vi "Build.Auto Build Manager.vi"(11 "App Build Spec":u16(ring) items=["Circle Test App", "Circle Test App Installer"]) -> (0 "Error":errorcluster, 3 "Build Ver":string)   [LabVIEW 2018]
uses:
  <vilib>/AppBuilder/AB_API_Simple/Get Build Specification Version (project reference).vi
  <vilib>/AppBuilder/AB_API_Simple/Build (project reference).vi
  <vilib>/Utility/config.llb/Write Key (Boolean).vi
  <vilib>/AppBuilder/AB_API_Simple/NI_App_Builder_API.lvlib
  <vilib>/KATE/Files/File Utils.lvlib
  <vilib>/Utility/config.llb/NI_LVConfig.lvlib
panel:
  in  "Proj List refresh":bool
  in  "Project":i32(ring) items=["Circle Test.lvproj"]
  out "MultInst":string
  in  "MultExe":bool caption="Allow Multiple Exe Instances"
  in  "Open Installer Folder":bool
  out "Found Installer":bool
  out "Status":string
  in  "Clear Error":bool
  in  "Exit":bool
  in  "Build":bool
  in  "Build Installer":bool=TRUE
  in  "Build App":bool=TRUE
  out "Building Installer":bool
  out "Building App":bool
  in  "Data Tab":T1(tab)
  out "App files":path[](array[path])
  out "Installer files":path[](array[path])
  out "New Path":path
  out "Orig Path":path
  out "BuildSpecs":string[](array[string])
  out "BuildDir":path
  out "BuildINI":path
  in  "Installer Build Spec":string
  # "App Builder"
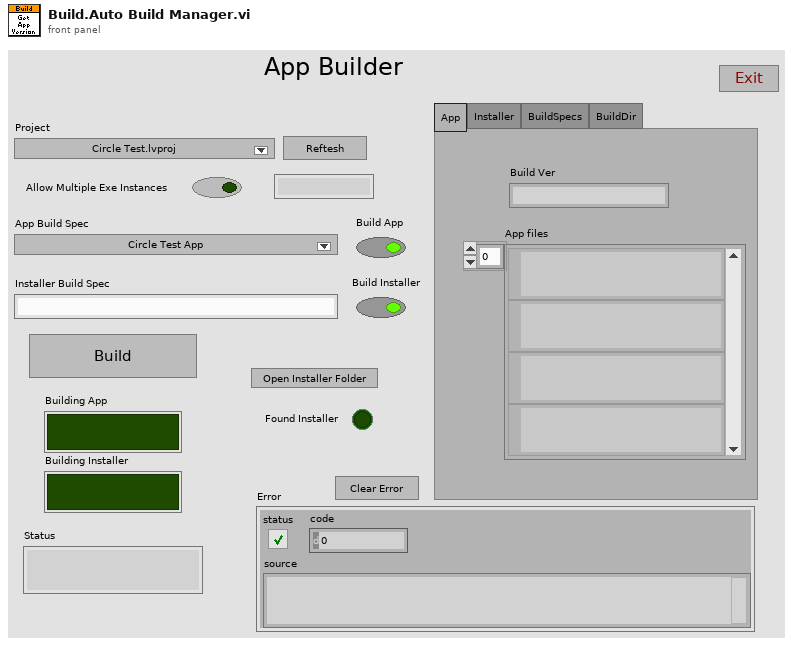
[diagram p1: front panel]
types:
  T1 = enum32{"App", "Installer", "BuildSpecs", "BuildDir"}
  T2 = cluster{"Proj":refnum<vi>, "Proj Name":string, "App Ver":string, "Installer":refnum<vi>, "Installer Name":string, "BuildSpec":refnum<vi>}
  T3 = typedef "NI_App_Builder_API.lvlib/Build Specification Version.ctl" = cluster{"Major":u16, "Minor":u16, "Fix":u16, "Build":u16}
  T4 = typedef "NI_LVConfig.lvlib/Config Data RefNum.ctl" = refnum<k1>
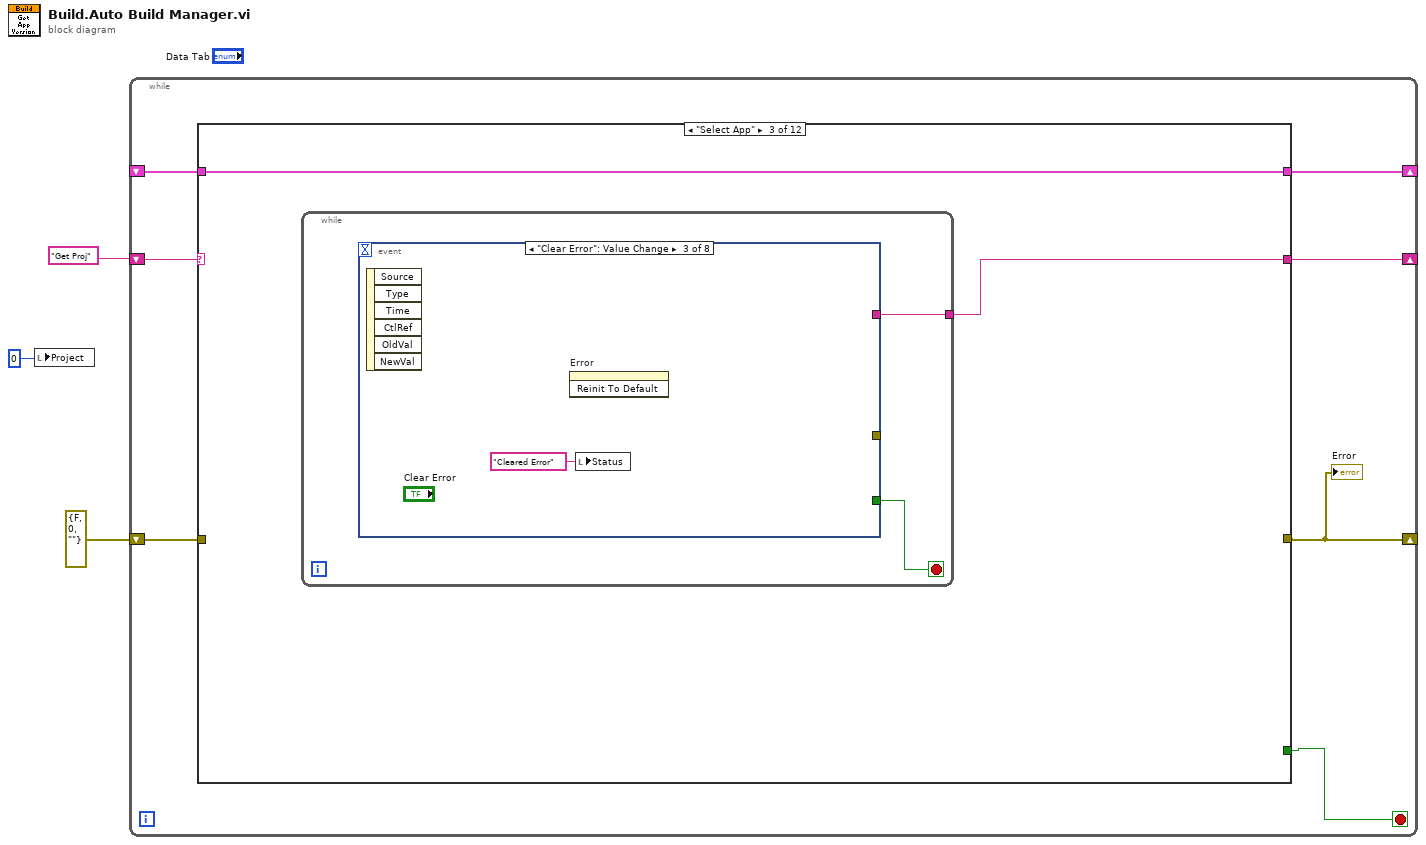
[diagram p0: block diagram]
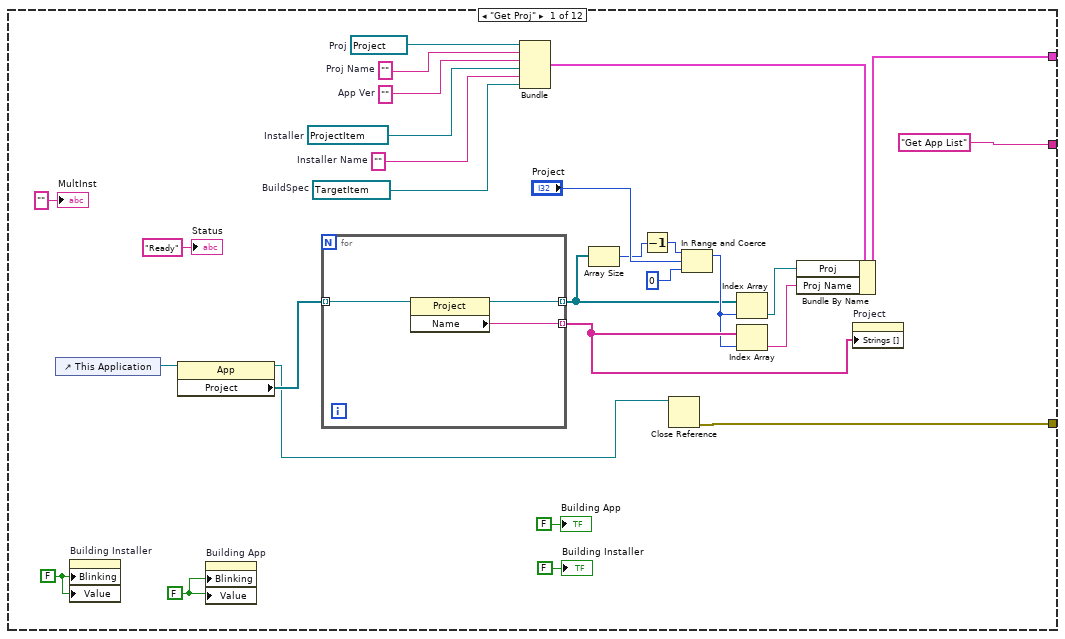
[diagram p2: hidden frame]
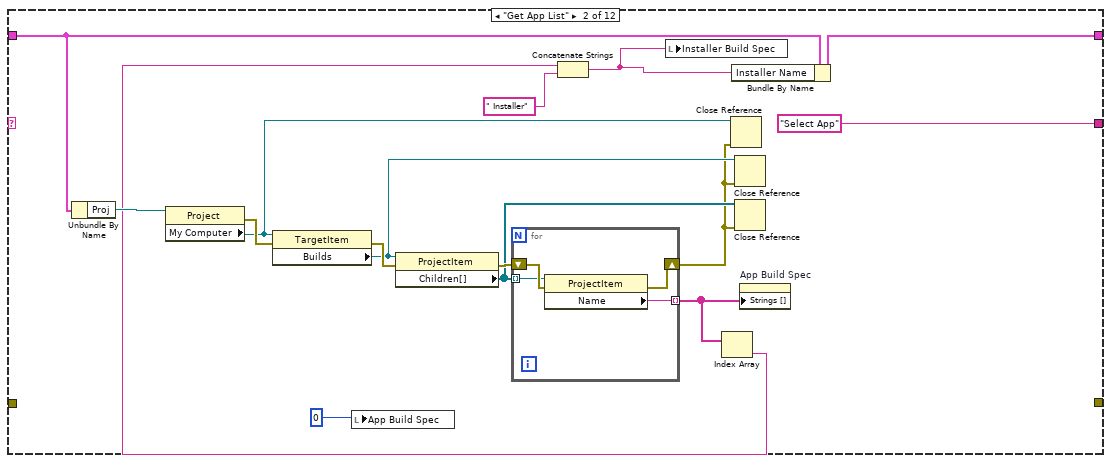
[diagram p3: hidden frame]
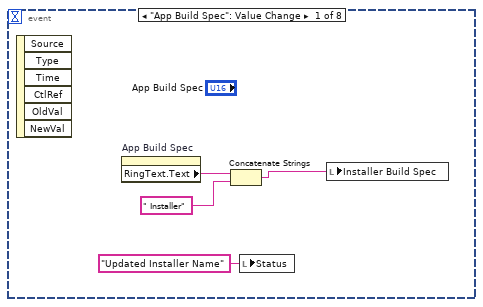
[diagram p4: hidden frame]
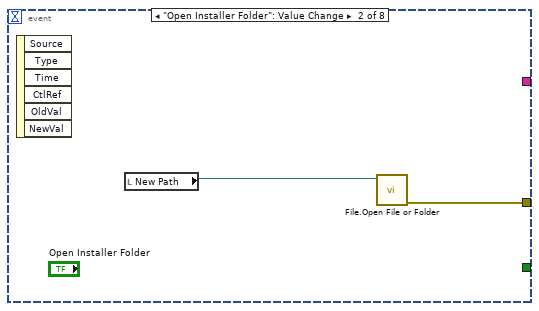
[diagram p5: hidden frame]
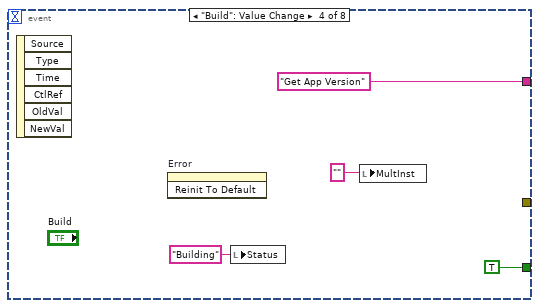
[diagram p6: hidden frame]
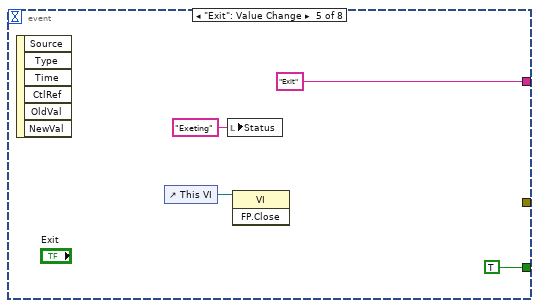
[diagram p7: hidden frame]
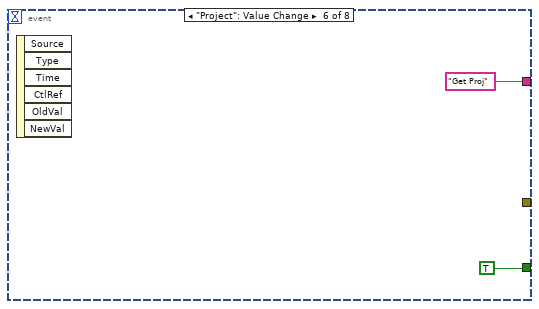
[diagram p8: hidden frame]
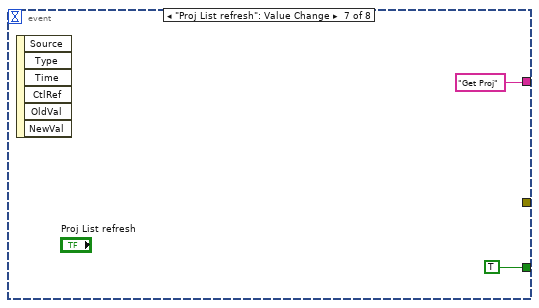
[diagram p9: hidden frame]
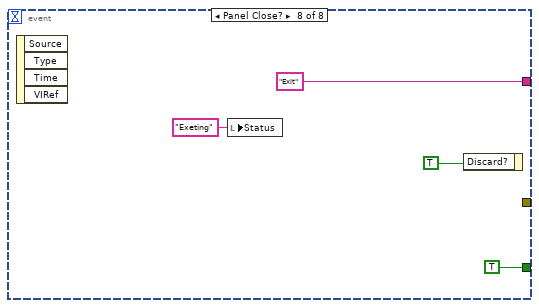
[diagram p10: hidden frame]
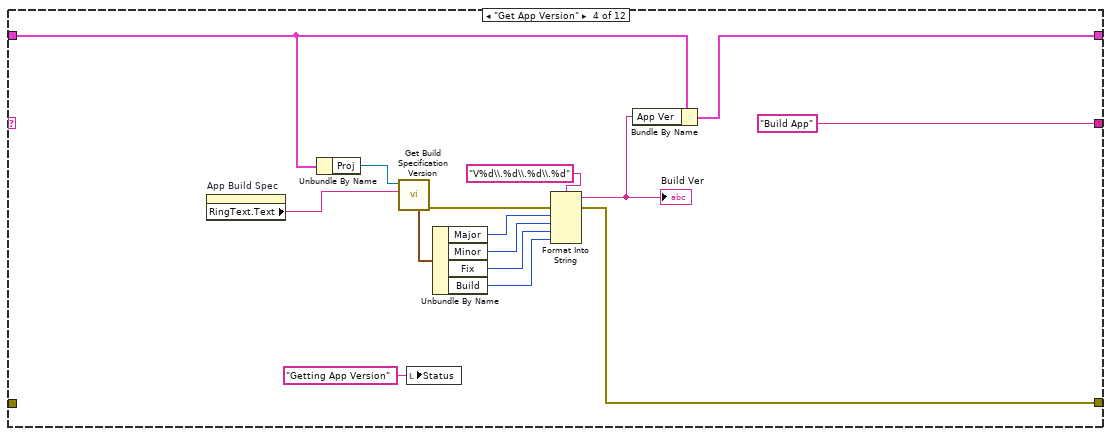
[diagram p11: hidden frame]
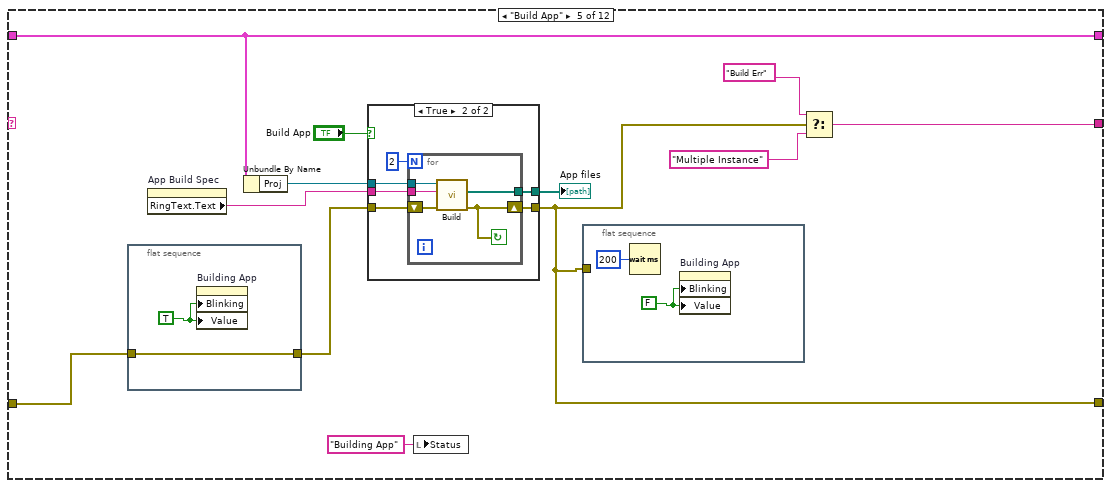
[diagram p12: hidden frame]
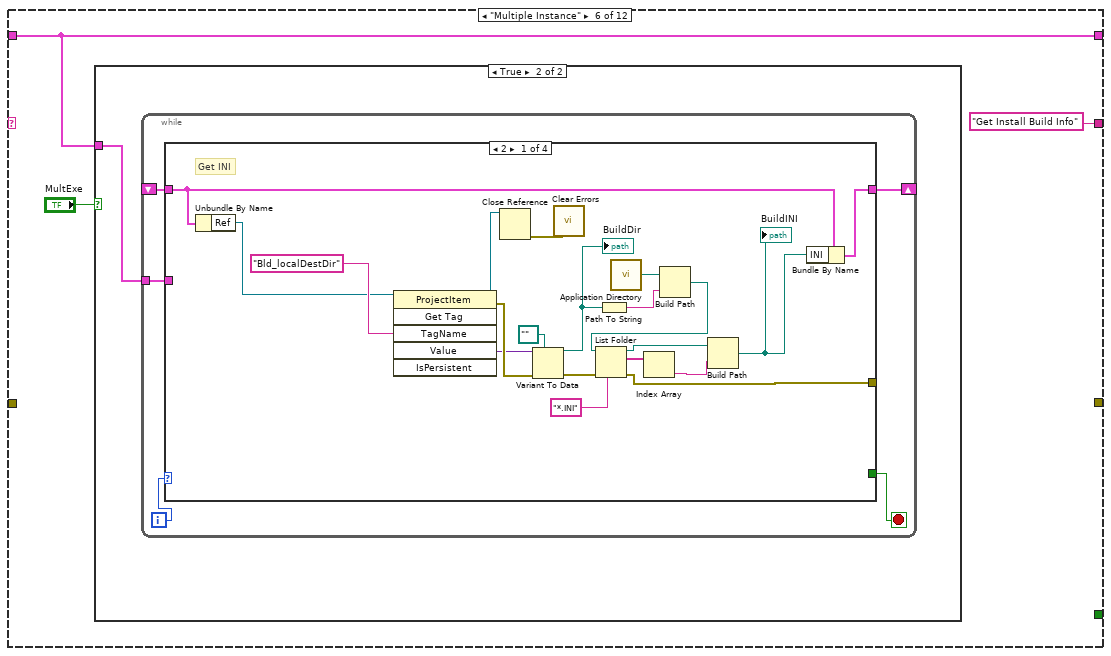
[diagram p14: hidden frame]
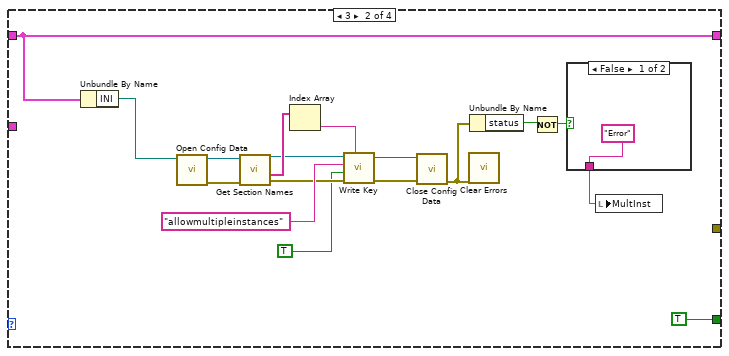
[diagram p16: hidden frame]
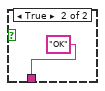
[diagram p17: hidden frame]
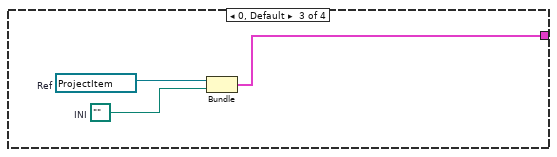
[diagram p18: hidden frame]
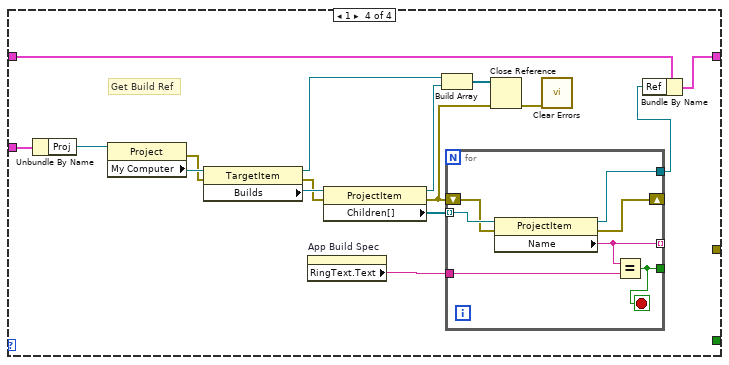
[diagram p19: hidden frame]
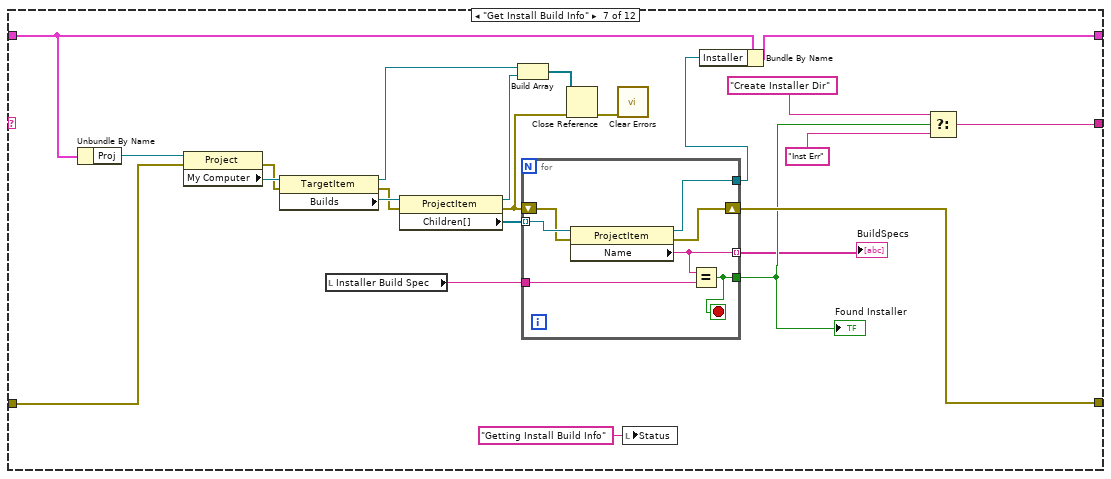
[diagram p20: hidden frame]
diagram:
  n1 = local write "Project"(0) -> ()
  n2 = while {
    shift-right: [w8] -> _
    shift-left: _ -> [w9]
    shift-right: [w7] -> _
    shift-left: "Get Proj" -> [w10]
    shift-right: [w5] -> _
    shift-left: errorcluster {"status"=FALSE, "code"=0, "source"=""} ("error constant") -> [w6]
    stop <- w4 stop-if-true
    n3 = case shown="\"Select App\"" w10 {
      tunnel: w9 -> [_ w44 w63 w95 w114 w132 w215 w238 w241 w256 w263 w284]
      tunnel: [w33 w43 w63 w93 w114 w132 w214 w238 w241 w256 w263 _] -> w8
      tunnel: ["Get App List" "Select App" w62 "Build App" w107 "Get Install Build Info" w210 "Select App" "Select App" "Build Installer" "Select App" _] -> w7
      tunnel: [w31 _ _ w89 w105 _ w221 errorcluster {"status"=TRUE, "code"=1, "source"="Installer not found.  Check Name."} ("error constant") errorcluster {"status"=TRUE, "code"=1, "source"="Build Error."} ("error constant") w242 w262 _] -> w5
      tunnel: w6 -> [_ _ _ _ w112 _ w224 _ _ _ _ _]
      tunnel: [_ _ _ _ _ _ _ _ _ _ _ TRUE] -> w4
      frame "Get Proj" {
        w22 = FALSE ("Building App")
        w23 = FALSE ("Blinking")
        w25 = refnum<vi> refnum  # BuildSpec
        w27 = refnum<vi> refnum  # Installer
        w28 = ""  # Installer Name
        w32 = ""  # App Ver
        w36 = refnum<vi> refnum  # Proj
        w37 = ""  # Proj Name
        n4 = control-ref of="This Application"() -> (w38:refnum<vi>)
        n5 = property on="Building Installer" class="Bool (strict)"("Blinking"=w23, "Value"=w23) -> ()  [unwired: 2 in, 2 out]
        n6 = property class="App"(reference=w38) -> (reference out=w20:refnum<vi>, "Project"=w21:refnum<vi>[])  [unwired: 1 in, 1 out]
        n7 = property on="Building App" class="Bool (strict)"("Blinking"=w22, "Value"=w22) -> ()  [unwired: 2 in, 2 out]
        n8 = for {
          tunnel: w21 -> [w41] mode=indexing
          tunnel: [w40] -> w17 mode=indexing
          tunnel: [w39] -> w14 mode=indexing
          n9 = property class="Project"(reference=w41) -> (reference out=w39:refnum<vi>, "Name"=w40:string)  [unwired: 1 in, 1 out]
        }
        n10 = Bundle("Proj"=w36, "Proj Name"=w37, "App Ver"=w32, "Installer"=w27, "Installer Name"=w28, "BuildSpec"=w25) -> (w34:T2)  [unwired: 1 in]
        n11 = Array Size(array=w14) -> (size(s)=w12:i32)
        n12 = Decrement(x=w12) -> (x-1=w11:i32)
        n13 = Close Reference(reference=w20) -> (error out=w31:errorcluster)  [unwired: 1 in]
        n14 = In Range and Coerce(upper limit=w11, x="Project", lower limit=0) -> (coerced(x)=w15:i32)  [unwired: 1 out]
        n15 = Index Array(array=w14, index=w15) -> (element=w19:refnum<vi>)
        n16 = Index Array(array=w17, index=w15) -> (element=w18:string)
        n17 = Bundle By Name(cluster=w34, "Proj"=w19, "Proj Name"=w18) -> (w33:T2)
        n18 = property on="Project" class="Ring (strict)"("Strings []"=w17) -> ()  [unwired: 2 in, 2 out]
        "Building App" <- FALSE ("Building App")
        "Building Installer" <- FALSE ("Building Installer")
        "Status" <- "Ready" ("Status")
        "MultInst" <- "" ("MultInst")
      }
      frame "Get App List" {
        n19 = Unbundle By Name(w44) -> ("Proj"=w57:refnum<vi>)
        n20 = property class="Project"(reference=w57) -> (error out=w56:errorcluster, "My Computer"=w51:refnum<vi>)  [unwired: 1 in, 1 out]
        n21 = property class="TargetItem"(reference=w51, error in=w56) -> (error out=w55:errorcluster, "Builds"=w52:refnum<vi>)  [unwired: 1 out]
        n22 = local write "App Build Spec"(u16 0) -> ()
        n23 = property class="ProjectItem"(reference=w52, error in=w55) -> (error out=w54:errorcluster, "Children[]"=w53:refnum<vi>[])  [unwired: 1 out]
        n24 = for {
          shift-right: [w59] -> w50
          shift-left: w54 -> [w61]
          tunnel: w53 -> [w60] mode=indexing
          tunnel: [w58] -> w48 mode=indexing
          n25 = property class="ProjectItem"(reference=w60, error in=w61) -> (error out=w59:errorcluster, "Name"=w58:string)  [unwired: 1 out]
        }
        n26 = Index Array(array=w48) -> (element=w46:string)  [unwired: 1 in]
        n27 = Concatenate Strings(w46, " Installer") -> (w42:string)
        n28 = local write "Installer Build Spec"(w42) -> ()
        n29 = Close Reference(reference=w51, error in (no error)=w50) -> ()  [unwired: 1 out]
        n30 = Bundle By Name(cluster=w44, "Installer Name"=w42) -> (w43:T2)
        n31 = Close Reference(reference=w52, error in (no error)=w50) -> ()  [unwired: 1 out]
        n32 = Close Reference(reference=w53, error in (no error)=w50) -> ()  [unwired: 1 out]
        n33 = property on="App Build Spec" class="Ring (strict)"("Strings []"=w48) -> ()  [unwired: 2 in, 2 out]
      }
      frame "Select App" {
        n34 = while {
          tunnel: [w65] -> w62
          stop <- w64 stop-if-true
          n35 = event shown="[2] \"Clear Error\": Value Change" {
            selector: _ -> [_ _ _ _ _ _ _ _]
            dyn-events: _ -> [_ _ _ _ _ _ _ _]
            timeout: _ -> [_ _ _ _ _ _ _ _]
            tunnel: [_ _ _ "Get App Version" "Exit" "Get Proj" "Get Proj" "Exit"] -> w65
            tunnel: [_ _ _ TRUE TRUE TRUE TRUE TRUE] -> w64
            tunnel: [_ w71 _ _ _ _ _ _] -> _
            event "App Build Spec": Value Change {
              n36 = event-data() -> ()  [unwired: 1 in, 6 out]
              n37 = property on="App Build Spec" class="Ring (strict)"() -> ("RingText.Text"=w69:string)  [unwired: 2 in, 2 out]
              n38 = Concatenate Strings(w69, " Installer") -> (w68:string)
              n39 = local write "Status"("Updated Installer Name" ("Status")) -> ()
              n40 = local write "Installer Build Spec"(w68) -> ()
            }
            event "Open Installer Folder": Value Change {
              n41 = event-data() -> ()  [unwired: 1 in, 6 out]
              n42 = local read "New Path"() -> (w70:path)
              n43 = call <vilib>:"File.Open File or Folder.vi"("Path"=w70) -> ("Error Out"=w71:errorcluster)  [unwired: 10 in]
            }
            event "Clear Error": Value Change {
              n44 = event-data() -> ()  [unwired: 1 in, 6 out]
              n45 = invoke on="Error" class="Clust (strict)" method="Reinit To Default"() -> ()  [unwired: 3 in, 3 out]
              n46 = local write "Status"("Cleared Error" ("Status")) -> ()
            }
            event "Build": Value Change {
              n47 = event-data() -> ()  [unwired: 1 in, 6 out]
              n48 = invoke on="Error" class="Clust (strict)" method="Reinit To Default"() -> ()  [unwired: 3 in, 3 out]
              n49 = local write "Status"("Building" ("Status")) -> ()
              n50 = local write "MultInst"("" ("MultInst")) -> ()
            }
            event "Exit": Value Change {
              n51 = event-data() -> ()  [unwired: 1 in, 6 out]
              n52 = control-ref of="This VI"() -> (w77:refnum<vi>)
              n53 = local write "Status"("Exeting" ("Status")) -> ()
              n54 = invoke class="VI" method="FP.Close"(reference=w77) -> ()  [unwired: 2 in, 3 out]
            }
            event "Project": Value Change {
              n55 = event-data() -> ()  [unwired: 1 in, 6 out]
            }
            event "Proj List refresh": Value Change {
              n56 = event-data() -> ()  [unwired: 1 in, 6 out]
            }
            event Panel Close? {
              n57 = event-data() -> ()  [unwired: 1 in, 4 out]
              n58 = local write "Status"("Exeting" ("Status")) -> ()
              n59 = event-data("Discard?"=TRUE) -> ()  [unwired: 1 in, 1 out]
            }
          }
        }
      }
      frame "Get App Version" {
        n60 = property on="App Build Spec" class="Ring (strict)"() -> ("RingText.Text"=w91:string)  [unwired: 2 in, 2 out]
        n61 = Unbundle By Name(w95) -> ("Proj"=w96:refnum<vi>)
        n62 = call-poly <vilib>:"Get Build Specification Version.vi"("Name of build specification"=w91, "Project reference"=w96) -> ("error out"=w103:errorcluster, "Build Specification Version"=w99:T3)  [unwired: 7 in, 1 out]
        n63 = local write "Status"("Getting App Version" ("Status")) -> ()
        n64 = Unbundle By Name(w99) -> ("Major"=w100:u16, "Minor"=w101:u16, "Fix"=w102:u16, "Build"=w97:u16)
        n65 = Format Into String(format string="V%d\\.%d\\.%d\\.%d", error in=w103, w100, w101, w102, w97) -> (resulting string=w94:string, error out=w89:errorcluster)  [unwired: 1 in]
        "Build Ver" <- w94
        n66 = Bundle By Name(cluster=w95, "App Ver"=w94) -> (w93:T2)
      }
      frame "Build App" {
        n67 = flat-sequence {
          tunnel: w112 -> [w130]
          tunnel: [w130] -> w111
          frame #0 {
            w131 = TRUE ("Building App")
            n68 = property on="Building App" class="Bool (strict)"("Blinking"=w131, "Value"=w131) -> ()  [unwired: 2 in, 2 out]
          }
        }
        n69 = property on="App Build Spec" class="Ring (strict)"() -> ("RingText.Text"=w109:string)  [unwired: 2 in, 2 out]
        n70 = Unbundle By Name(w114) -> ("Proj"=w115:refnum<vi>)
        n71 = case shown="True" "Build App" {
          tunnel: w115 -> [_ w122]
          tunnel: w109 -> [_ w121]
          tunnel: [_ w120] -> w113
          tunnel: [w116 w119] -> w105
          tunnel: w111 -> [w116 w118]
          frame False {
          }
          frame True {
            n72 = for {
              N: 2 -> [_]
              tunnel: w122 -> [w127]
              tunnel: w121 -> [w126]
              tunnel: [w125] -> w120
              shift-right: [w123] -> w119
              shift-left: w118 -> [w124]
              stop <- w123 continue-if-true
              n73 = call-poly <vilib>:"Build.vi"("error in (no error)"=w124, "Name of build specification (if empty: build all)"=w126, "Project reference"=w127) -> ("error out"=w123:errorcluster, "Generated files"=w125:path[])  [unwired: 6 in, 1 out]
            }
          }
        }
        "App files" <- w113
        n74 = local write "Status"("Building App" ("Status")) -> ()
        n75 = flat-sequence {
          tunnel: w105 -> [_]
          frame #0 {
            w129 = FALSE ("Building App")
            n76 = Wait (ms)(milliseconds to wait=u32 200) -> ()  [unwired: 1 out]
            n77 = property on="Building App" class="Bool (strict)"("Blinking"=w129, "Value"=w129) -> ()  [unwired: 2 in, 2 out]
          }
        }
        n78 = Select(t="Build Err", s=w105, f="Multiple Instance") -> (s? t:f=w107:string)
      }
      frame "Multiple Instance" {
        n79 = case shown="True" "MultExe" {
          tunnel: w132 -> [_ w135]
          frame False {
          }
          frame True {
            n80 = while {
              shift-right: [w140] -> _
              shift-left: _ -> [w138]
              tunnel: w135 -> [w136]
              i -> [w139]
              stop <- w137 stop-if-true
              n81 = case shown="2" w139 {
                tunnel: [w149 w166 w180 w185] -> w140
                tunnel: w138 -> [w150 w166 _ w186]
                tunnel: [_ TRUE _ _] -> w137
                tunnel: w136 -> [_ _ _ w184]
                tunnel: [w147 _ _ _] -> _
                frame 2 {
                  # "Get INI"
                  n82 = Unbundle By Name(w150) -> ("Ref"=w152:refnum<vi>)
                  n83 = invoke class="ProjectItem" method="Get Tag"(reference=w152, "TagName"="Bld_localDestDir") -> (reference out=w145:refnum<vi>, error out=w160:errorcluster, "Value"=w159:variant)  [unwired: 4 in, 3 out]
                  n84 = Close Reference(reference=w145) -> (error out=w151:errorcluster)  [unwired: 1 in]
                  n85 = Variant To Data(error in=w160, type=path "", Variant=w159) -> (data=w143:path, error out=w148:errorcluster)
                  "BuildDir" <- w143
                  n86 = call <vilib>:"Clear Errors.vi"("error in (no error)"=w151) -> ()  [unwired: 5 in, 2 out]
                  n87 = Path To String(path=w143) -> (string=w142:string)
                  n88 = call <vilib>:"Application Directory.vi"() -> ("Application Directory"=w144:path)
                  n89 = Build Path(base path=w144, name or relative path=w142) -> (appended path=w141:path)
                  n90 = List Folder(path=w141, pattern="*.INI", error in=w148) -> (path out=w154:path, filenames=w155:string[], error out=w147:errorcluster)  [unwired: 1 in, 1 out]
                  n91 = Index Array(array=w155) -> (element=w153:string)  [unwired: 1 in]
                  n92 = Build Path(base path=w154, name or relative path=w153) -> (appended path=w146:path)
                  "BuildINI" <- w146
                  n93 = Bundle By Name(cluster=w150, "INI"=w146) -> (w149:cluster{"Ref":refnum<vi>, "INI":path})
                }
                frame 3 {
                  n94 = Unbundle By Name(w166) -> ("INI"=w176:path)
                  n95 = call <vilib>:"Open Config Data.vi"("configuration file path"=w176) -> ("error out"=w175:errorcluster, "refnum"=w177:T4)  [unwired: 8 in, 1 out]
                  n96 = call <vilib>:"Get Section Names.vi"("error in (no error)"=w175, "refnum"=w177) -> ("error out"=w170:errorcluster, "section names"=w174:string[], "refnum out"=w173:T4)  [unwired: 7 in]
                  n97 = Index Array(array=w174) -> (element=w172:string)  [unwired: 1 in]
                  n98 = call-poly <vilib>:"Write Key.vi"("section"=w172, "error in (no error)"=w170, "value"=TRUE, "key"="allowmultipleinstances", "refnum"=w173) -> ("error out"=w167:errorcluster, "refnum out"=w168:T4)  [unwired: 4 in, 1 out]
                  n99 = call <vilib>:"Close Config Data.vi"("error in (no error)"=w167, "refnum"=w168) -> ("error out"=w164:errorcluster)  [unwired: 8 in, 1 out]
                  n100 = call <vilib>:"Clear Errors.vi"("error in (no error)"=w164) -> ()  [unwired: 5 in, 2 out]
                  n101 = Unbundle By Name(w164) -> ("status"=w163:bool)
                  n102 = Not(x=w163) -> (.not. x?=w162:bool)
                  n103 = case shown="False" w162 {
                    tunnel: ["Error" "OK"] -> w161
                    frame False {
                    }
                    frame True {
                    }
                  }
                  n104 = local write "MultInst"(w161) -> ()
                }
                frame 0, Default {
                  w181 = path ""  # INI
                  w182 = refnum<vi> refnum  # Ref
                  n105 = Bundle("Ref"=w182, "INI"=w181) -> (w180:cluster{"Ref":refnum<vi>, "INI":path})  [unwired: 1 in]
                }
                frame 1 {
                  # "Get Build Ref"
                  n106 = Unbundle By Name(w184) -> ("Proj"=w198:refnum<vi>)
                  n107 = property class="Project"(reference=w198) -> (error out=w194:errorcluster, "My Computer"=w197:refnum<vi>)  [unwired: 1 in, 1 out]
                  n108 = property class="TargetItem"(reference=w197, error in=w194) -> (reference out=w192:refnum<vi>, error out=w193:errorcluster, "Builds"=w196:refnum<vi>)
                  n109 = property on="App Build Spec" class="Ring (strict)"() -> ("RingText.Text"=w187:string)  [unwired: 2 in, 2 out]
                  n110 = property class="ProjectItem"(reference=w196, error in=w193) -> (reference out=w191:refnum<vi>, error out=w188:errorcluster, "Children[]"=w195:refnum<vi>[])
                  n111 = Build Array(w192, w191) -> (w190:refnum<vi>[])
                  n112 = for {
                    tunnel: w195 -> [w205] mode=indexing
                    shift-right: [w203] -> _
                    shift-left: w188 -> [w204]
                    tunnel: [w202] -> w183
                    tunnel: [w201] -> _
                    tunnel: [w200] -> _ mode=indexing
                    tunnel: w187 -> [w199]
                    stop <- w201 stop-if-true
                    n113 = property class="ProjectItem"(reference=w205, error in=w204) -> (reference out=w202:refnum<vi>, error out=w203:errorcluster, "Name"=w200:string)
                    n114 = Equal?(x=w200, y=w199) -> (x = y?=w201:bool)
                  }
                  n115 = Close Reference(reference=w190, error in (no error)=w188) -> (error out=w189:errorcluster)
                  n116 = call <vilib>:"Clear Errors.vi"("error in (no error)"=w189) -> ()  [unwired: 5 in, 2 out]
                  n117 = Bundle By Name(cluster=w186, "Ref"=w183) -> (w185:cluster{"Ref":refnum<vi>, "INI":path})
                }
              }
            }
          }
        }
      }
      frame "Get Install Build Info" {
        n118 = Unbundle By Name(w215) -> ("Proj"=w228:refnum<vi>)
        n119 = property class="Project"(reference=w228, error in=w224) -> (error out=w223:errorcluster, "My Computer"=w227:refnum<vi>)  [unwired: 1 out]
        n120 = property class="TargetItem"(reference=w227, error in=w223) -> (reference out=w220:refnum<vi>, error out=w222:errorcluster, "Builds"=w226:refnum<vi>)
        n121 = local read "Installer Build Spec"() -> (w207:string)
        n122 = property class="ProjectItem"(reference=w226, error in=w222) -> (reference out=w219:refnum<vi>, error out=w216:errorcluster, "Children[]"=w225:refnum<vi>[])
        n123 = Build Array(w220, w219) -> (w218:refnum<vi>[])
        n124 = for {
          tunnel: w225 -> [w235] mode=indexing
          shift-right: [w233] -> w221
          shift-left: w216 -> [w234]
          tunnel: w207 -> [w232]
          tunnel: [w231] -> w213
          tunnel: [w230] -> w209
          tunnel: [w229] -> w206 mode=indexing
          stop <- w230 stop-if-true
          n125 = property class="ProjectItem"(reference=w235, error in=w234) -> (reference out=w231:refnum<vi>, error out=w233:errorcluster, "Name"=w229:string)
          n126 = Equal?(x=w229, y=w232) -> (x = y?=w230:bool)
        }
        "Found Installer" <- w209
        "BuildSpecs" <- w206
        n127 = Close Reference(reference=w218, error in (no error)=w216) -> (error out=w217:errorcluster)
        n128 = call <vilib>:"Clear Errors.vi"("error in (no error)"=w217) -> ()  [unwired: 5 in, 2 out]
        n129 = local write "Status"("Getting Install Build Info" ("Status")) -> ()
        n130 = Bundle By Name(cluster=w215, "Installer"=w213) -> (w214:T2)
        n131 = Select(t="Create Installer Dir", s=w209, f="Inst Err") -> (s? t:f=w210:string)
      }
      frame "Inst Err" {
      }
      frame "Build Err" {
      }
      frame "Create Installer Dir" {
        w252 = "INST_buildLocation"
        n132 = Unbundle By Name(w256) -> ("Installer"=w259:refnum<vi>)
        n133 = Unbundle By Name(w256) -> ("App Ver"=w254:string)
        n134 = invoke class="ProjectItem" method="Get Tag"(reference=w259, "TagName"=w252) -> (reference out=w253:refnum<vi>, error out=w249:errorcluster, "Value"=w247:variant)  [unwired: 4 in, 3 out]
        n135 = Variant To Data(error in=w249, type=path "", Variant=w247) -> (data=w257:path, error out=w248:errorcluster)
        "Orig Path" <- w257
        n136 = local write "Status"("Creating Install Folder" ("Status")) -> ()
        n137 = Strip Path(path=w257) -> (stripped path=w255:path)  [unwired: 1 out]
        n138 = Build Path(base path=w255, name or relative path=w254) -> (appended path=w246:path)
        n139 = call <vilib>:"File.Create Folder if Does Not Exist.vi"("Path"=w246) -> ("error out"=w244:errorcluster, "Dup Path"=→"New Path":path)  [unwired: 8 in, 1 out]
        n140 = invoke class="ProjectItem" method="Set Tag"(reference=w253, error in=w248, "TagName"=w252, "Value"=w246, "IsPersistent"=FALSE ("Is Persistent")) -> (error out=w243:errorcluster)  [unwired: 1 in, 5 out]
        n141 = Merge Errors(w243, w244) -> (w242:errorcluster)
      }
      frame "Build Installer" {
        n142 = flat-sequence {
          tunnel: w263 -> [w269]
          tunnel: [w268] -> w262
          tunnel: "Build Installer" -> [w267]
          frame #0 {
            w266 = TRUE ("Blinking")
            n143 = property on="Building Installer" class="Bool (strict)"("Blinking"=w266, "Value"=w266) -> ()  [unwired: 2 in, 2 out]
            n144 = local write "Status"("Building Installer" ("Status")) -> ()
          }
          frame #1 {
            n145 = case shown="True" w267 {
              tunnel: w269 -> [_ w275]
              tunnel: [_ w272] -> w268
              frame False {
              }
              frame True {
                n146 = Unbundle By Name(w275) -> ("Proj"=w274:refnum<vi>)
                n147 = for {
                  N: 2 -> [_]
                  tunnel: w274 -> [w279]
                  tunnel: [w278] -> w273
                  tunnel: [w276] -> w272
                  tunnel: "Installer Build Spec" -> [w277]
                  stop <- w276 continue-if-true
                  n148 = call-poly <vilib>:"Build.vi"("Name of build specification (if empty: build all)"=w277, "Project reference"=w279) -> ("error out"=w276:errorcluster, "Generated files"=w278:path[])  [unwired: 7 in, 1 out]
                }
                "Installer files" <- w273
              }
            }
          }
          frame #2 {
            w281 = FALSE ("Blinking")
            n149 = property on="Building Installer" class="Bool (strict)"("Blinking"=w281, "Value"=w281) -> ()  [unwired: 2 in, 2 out]
            n150 = local write "Status"("Done" ("Status")) -> ()
          }
        }
      }
      frame "Exit", Default {
        n151 = Unbundle By Name(w284) -> ("Proj"=w283:refnum<vi>)
        n152 = Close Reference(reference=w283) -> (error out=w282:errorcluster)  [unwired: 1 in]
        n153 = call <vilib>:"Clear Errors.vi"("error in (no error)"=w282) -> ()  [unwired: 5 in, 2 out]
      }
    }
    "Error" <- w5
  }
